vi "JSON Lookahead.vi"(8 "error in (no error)":errorcluster, 11 "Alpaca CLI Parser in":refnum<class "JSON Parser.lvclass">) -> (0 "error out":errorcluster, 1 "Lookahead Value":string, 2 "Lookahead Type":T1=enum."comma", 3 "Alpaca CLI Parser out":refnum<class "JSON Parser.lvclass">)   [LabVIEW 2019, in "JKI JSON Serialization.lvlib" / "JSON Parser.lvclass"]
doc: "JKI JSON 1.1.10.37\nTomi Maila - JKI\nCopyright (c) 2017, JKI"
uses:
  JSON Parser.lvclass
  C:/Users/Patrick/Documents/GitHub/Instrument-Framework/lvsrc/SMOs/JSON-RPC-2019/lv-venv/lv.lib/vi.lib/addons/_JKI.lib/Serialization/JSON/Deserializer/Parser/Parser.lvclass
  JSON Lexer/JSON Token Type.ctl
  Parser/Parser.lvclass/Parser.ctl
  JSON Lexer/JSON Lexer.lvclass
  Parser/Parser.lvclass
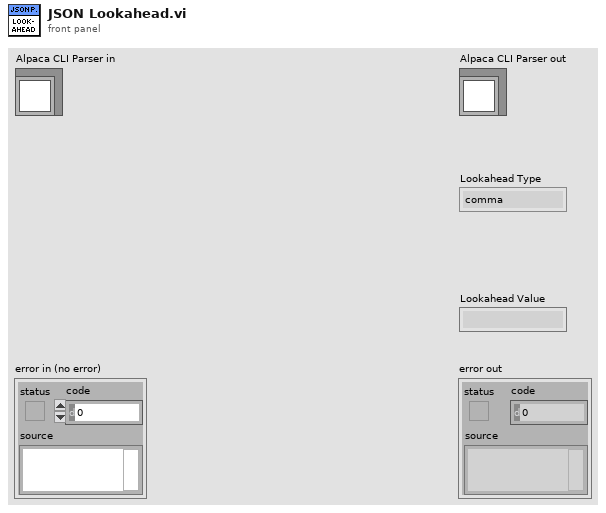
[diagram p1: front panel]
types:
  T1 = typedef "JKI JSON Serialization.lvlib/JSON Lexer.lvclass/JSON Token Type.ctl" = enum32{"unknown", "comma", "end-label", "begin-object", "end-object", "begin-array", "end-array", "quoted-string", "boolean", "exponential-number", "decimal-number", "integer-number", "special-number", "null", "symbol", "whitespace", "EOF"}
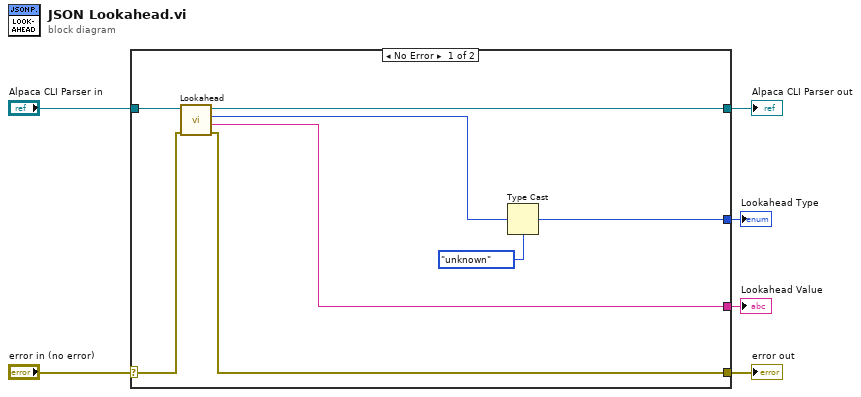
[diagram p0: block diagram]
diagram:
  n1 = case shown="No Error" "error in (no error)" {
    selector: "error in (no error)" -> [w7 w16]
    tunnel: [w8 w16] -> w5
    tunnel: [w11 w15] -> w3
    tunnel: "Alpaca CLI Parser in" -> [w12 w15]
    tunnel: [w9 _] -> w2
    tunnel: [w13 _] -> w1
    frame No Error {
      n2 = call "Lookahead.vi"("error in (no error)"=w7, "Alpaca Parser in"=w12) -> ("error out"=w8:errorcluster, "Lookahead Value"=w9:string, "Lookahead Type"=w10:i32, "Alpaca Parser out"=w11:refnum<class "JSON Parser.lvclass">)  [unwired: 6 in]
      n3 = Type Cast(type=JSON_Token_Type."unknown" ("CLI Token"), x=w10) -> (*(type *) &x=w13:T1)
    }
    frame Error {
    }
  }
  "error out" <- w5
  "Alpaca CLI Parser out" <- w3
  "Lookahead Type" <- w1
  "Lookahead Value" <- w2
